vi "TimeLapse save images.vi"(7 "Logging queue":refnum<queue>, 8 "error in (no error)":errorcluster, 9 "Ch1-Green":i16[][](array[numeric]), 10 "Ch0-Red":i16[][](array[numeric]), 11 "Logging queue element":T1={"Imaging Protocol"=enum."Live Imaging", "Number of Trials"=0, "Frame Size"=512, "# Averaged frames"=0, "Dwell time (us)"=0.0, "Index of Z-plane"=0, "Timelapse?"=FALSE, "Logging process is active"=FALSE, "Speed logging enabled"=FALSE, "tdms file ref"=refnum, "path"=path "", "Trial Number"=0, "Expected # points acquired"=FALSE, "Manually stopped"=FALSE, "Ch0 data"=[], "Ch1 data"=[], "Last trial"=FALSE, "Points acquired"={"Ch0 last trial"=0, "Ch1 last trial"=0, "All trials"=0}} {"Frame Size" items=["100X100"=100, "128X128"=128, "200X200"=200, "256X256"=256, "512X512"=512, "1024x1024"=1024, "2048x2048"=2048]; "Dwell time (us)" format="%#.6g"}) -> (0 "error":errorcluster)   [LabVIEW 2013]
uses:
  Typedefs/Logging queue element.ctl
  Typedefs/Imaging Protocols enum.ctl
  Typedefs/Frame Size.ctl
  Typedefs/Acquired points count.ctl
  Typedefs/Channel Selector.ctl
  Typedefs/Top level VI states.ctl
  Global Variables/General Globals.vi
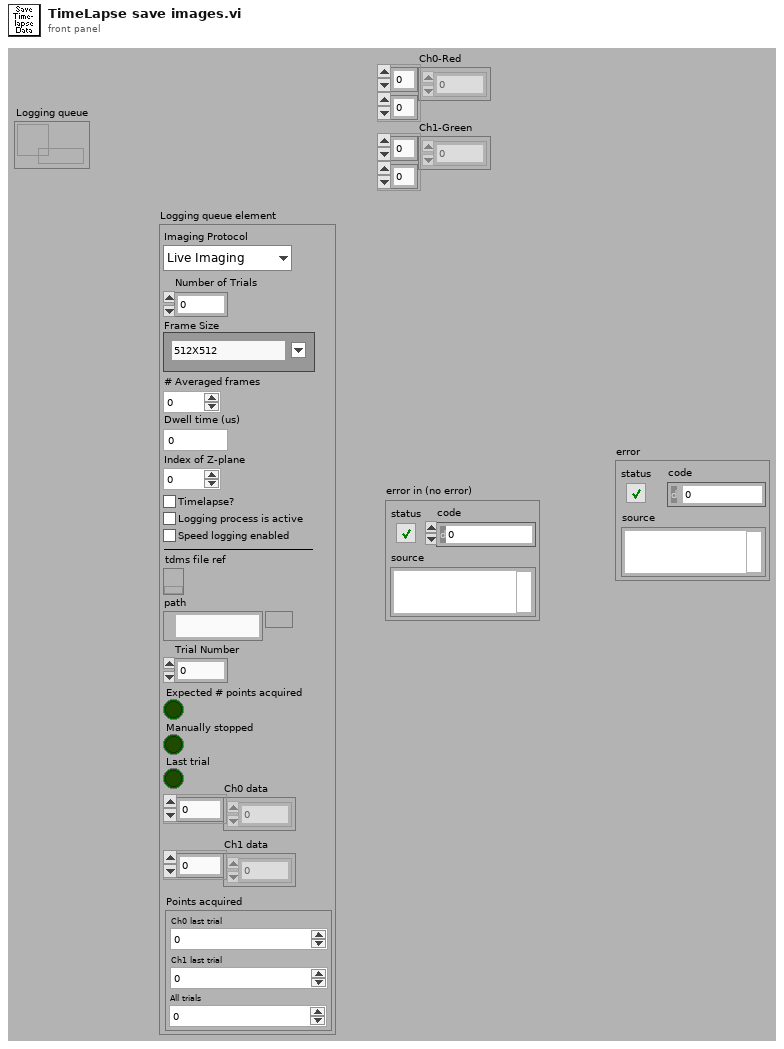
[diagram p1: front panel]
types:
  T1 = typedef "Logging queue element.ctl" = cluster{"Imaging Protocol":T2, "Number of Trials":u16, "Frame Size":T3, "# Averaged frames":u16, "Dwell time (us)":dbl, "Index of Z-plane":i32, "Timelapse?":bool, "Logging process is active":bool, "Speed logging enabled":bool, "tdms file ref":refnum<k34>, "path":path, "Trial Number":i32, "Expected # points acquired":bool, "Manually stopped":bool, "Ch0 data":u32[], "Ch1 data":u32[], "Last trial":bool, "Points acquired":T4}
  T2 = typedef "Imaging Protocols enum.ctl" = enum16{"AOL Z-Stack", "Motor Z Stack", "Functional Acquisition", "Single Plane Acquisition", "Volume Acquisition", "Live Imaging", "Live Plane Imaging", "Live Volume Imaging"}
  T3 = typedef "Frame Size.ctl" = u16
  T4 = typedef "Acquired points count.ctl" = cluster{"Ch0 last trial":u64, "Ch1 last trial":u64, "All trials":u64}
  T5 = typedef "Channel Selector.ctl" = enum16{"Red Channel", "Green Channel", "Blended"}
  T6 = typedef "Top level VI states.ctl" = enum16{"None", "Initialise UI", "<STACK PROTOCOL STATES>", "AOL Zstack-START", "AOL Zstack-STOP", "Motor Zstack-START", "Motor Zstack-STOP", "<ACQUISITION PROTOCOL STATES> ", "Functional Acquisition-START", "Functional Acquisition-STOP", "Single Plane Acquisition-START", "Single Plane Acquisition-STOP", "Volume Acquisition-START", "Volume Acquisition-STOP", "<LIVE IMAGING PROTOCOL STATES>", "Live Imaging-START", "Live Imaging-STOP", "Live Plane Imaging-START", "Live Plane Imaging-STOP", "Live Volume Imaging-START", "Live Volume Imaging-STOP", "EXIT"}
  T7 = typedef "AVI implementation enum.ctl" = enum16{"AVI1", "AVI2"}
  T8 = typedef "AVI Refs cluster.ctl" = cluster{"AVI2 path":path, "AVI 2 Refnum":T9, "New Image":T10, "error out":errorcluster, "Avi 1 Refnum":T11}
  T9 = typedef "IMAQ AVI2 Refnum.ctl" = refnum<k20>
  T10 = typedef "IMAQ Image.ctl" = refnum<image>
  T11 = typedef "AviRefnum.ctl" = refnum<k1>
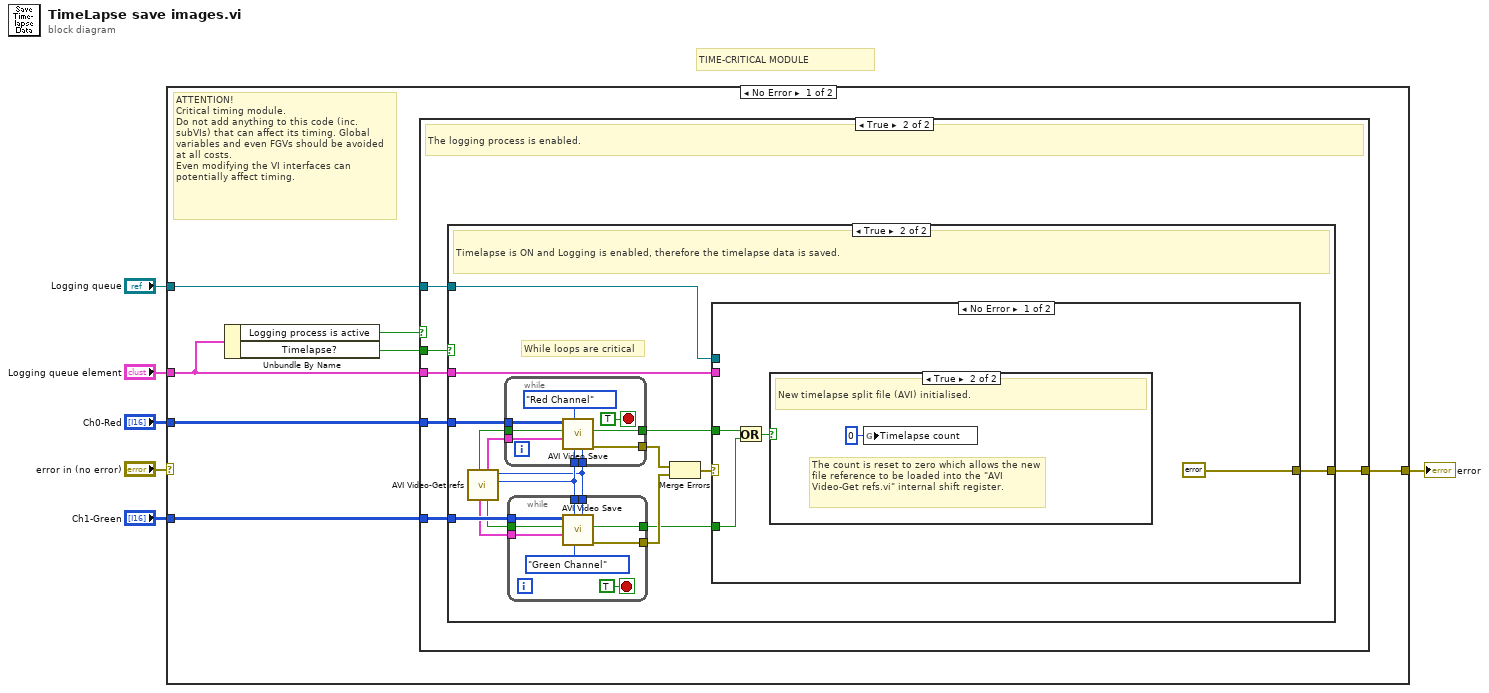
[diagram p0: block diagram]
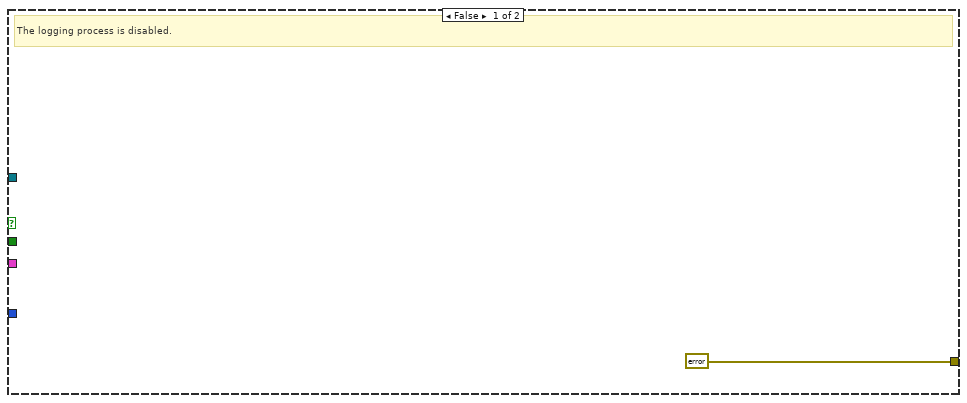
[diagram p2: hidden frame]
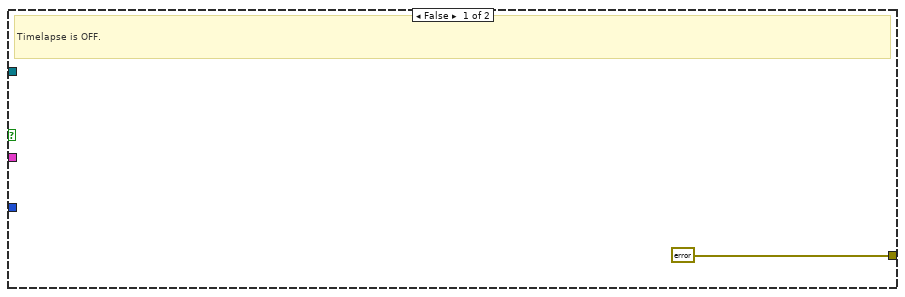
[diagram p3: hidden frame]
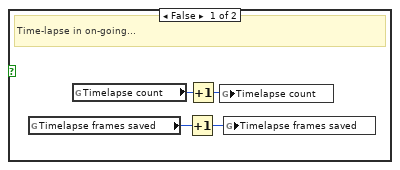
[diagram p4: hidden frame]
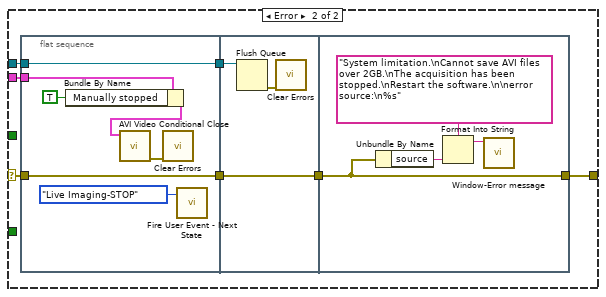
[diagram p5: hidden frame]
diagram:
  # "TIME-CRITICAL MODULE"
  n1 = case shown="No Error" "error in (no error)" {
    selector: "error in (no error)" -> [_ w86]
    tunnel: [w13 w86] -> w6
    tunnel: "Logging queue element" -> [w8 _]
    tunnel: "Ch0-Red" -> [w12 _]
    tunnel: "Ch1-Green" -> [w11 _]
    tunnel: "Logging queue" -> [w9 _]
    frame No Error {
      # "ATTENTION!\nCritical timing module.\nDo not add anything to this code (inc. subVIs) that can affect its timing. Global variables and even FGVs should be avoided at all costs.\nEven modifying the VI interfaces can potentially affect timing."
      n2 = Unbundle By Name(w8) -> ("Logging process is active"=w7:bool, "Timelapse?"=w10:bool)
      n3 = case shown="True" w7 {
        tunnel: [errorcluster {"status"=FALSE, "code"=0, "source"=""} ("error IO") w20] -> w13
        tunnel: w12 -> [_ w19]
        tunnel: w11 -> [_ w18]
        tunnel: w10 -> [_ w17]
        tunnel: w8 -> [_ w16]
        tunnel: w9 -> [_ w15]
        frame False {
          # "The logging process is disabled."
        }
        frame True {
          # "The logging process is enabled."
          n4 = case shown="True" w17 {
            tunnel: [errorcluster {"status"=FALSE, "code"=0, "source"=""} ("error IO") w26] -> w20
            tunnel: w19 -> [_ w35]
            tunnel: w18 -> [_ w34]
            tunnel: w16 -> [_ w28]
            tunnel: w15 -> [_ w27]
            frame False {
              # "Timelapse is OFF."
            }
            frame True {
              # "While loops are critical"
              # "Timelapse is ON and Logging is enabled, therefore the timelapse data is saved."
              n5 = call "AVI Video-Get refs.vi"() -> ("AVI mode"=w29:T7, "Frame Size"=w22:u32, "Green PMT is ON"=w31:bool, "Red AVI"=w32:T8, "Green AVI"=w30:T8, "Red PMT is ON"=w33:bool)  [unwired: 5 in, 1 out]
              n6 = while {
                tunnel: [w55] -> w36
                tunnel: w35 -> [w54]
                tunnel: w33 -> [w53]
                tunnel: w32 -> [w52]
                tunnel: w29 -> [w51]
                tunnel: [w49] -> w23
                tunnel: w22 -> [w48]
                stop <- TRUE stop-if-true
                n7 = call "AVI Video Save.vi"("Frame Size"=w48, "Channel"=Channel_Selector."Red Channel", "AVI mode"=w51, "AVI cluster"=w52, "PMT is ON?"=w53, "Image Pixels"=w54) -> ("error out"=w55:errorcluster, "New split file has just been initialised"=w49:bool)  [unwired: 4 in]
              }
              n8 = while {
                tunnel: [w46] -> w37
                tunnel: w34 -> [w45]
                tunnel: w31 -> [w44]
                tunnel: w30 -> [w43]
                tunnel: w29 -> [w42]
                tunnel: [w40] -> w24
                tunnel: w22 -> [w39]
                stop <- TRUE stop-if-true
                n9 = call "AVI Video Save.vi"("Frame Size"=w39, "Channel"=Channel_Selector."Green Channel", "AVI mode"=w42, "AVI cluster"=w43, "PMT is ON?"=w44, "Image Pixels"=w45) -> ("error out"=w46:errorcluster, "New split file has just been initialised"=w40:bool)  [unwired: 4 in]
              }
              n10 = Merge Errors(w36, w37) -> (w25:errorcluster)
              n11 = case shown="No Error" w25 {
                selector: w25 -> [_ w66]
                tunnel: w28 -> [_ w71]
                tunnel: w27 -> [_ w70]
                tunnel: [errorcluster {"status"=FALSE, "code"=0, "source"=""} ("error IO") w65] -> w26
                tunnel: w24 -> [w58 _]
                tunnel: w23 -> [w59 _]
                frame No Error {
                  n12 = Or(x=w59, y=w58) -> (x .or. y?=w57:bool)
                  n13 = case shown="True" w57 {
                    frame False {
                      # "Time-lapse in on-going..."
                      n14 = global read "General Globals.vi" "Timelapse frames saved"() -> (w61:u32)
                      n15 = global read "General Globals.vi" "Timelapse count"() -> (w62:u32)
                      n16 = Increment(x=w61) -> (x+1=w60:u32)
                      n17 = Increment(x=w62) -> (x+1=w63:u32)
                      n18 = global write "General Globals.vi" "Timelapse count"(w63) -> ()
                      n19 = global write "General Globals.vi" "Timelapse frames saved"(w60) -> ()
                    }
                    frame True {
                      # "The count is reset to zero which allows the new file reference to be loaded into the \"AVI Video-Get refs.vi\" internal shift register."
                      # "New timelapse split file (AVI) initialised."
                      n20 = global write "General Globals.vi" "Timelapse count"(u32 0 ("Timelapse count")) -> ()
                    }
                  }
                }
                frame Error {
                  n21 = flat-sequence {
                    tunnel: w71 -> [w77]
                    tunnel: [w74] -> w69
                    tunnel: w70 -> [w74]
                    tunnel: [w72] -> w67
                    tunnel: w66 -> [w72]
                    tunnel: w69 -> [w80]
                    tunnel: [w79] -> w68
                    tunnel: w67 -> [w79]
                    tunnel: w68 -> [w82]
                    tunnel: [w82] -> w65
                    frame #0 {
                      n22 = Bundle By Name(cluster=w77, "Manually stopped"=TRUE) -> (w75:T1)
                      n23 = call "AVI Video Conditional Close.vi"("Logging queue element in"=w75) -> ("error out"=w78:errorcluster)  [unwired: 10 in]
                      n24 = call <vilib>:"Clear Errors.vi"("error in (no error)"=w78) -> ()  [unwired: 6 in, 1 out]
                      n25 = call "Fire User Event - Next State.vi"("\"UI Handler loop\" case to execute"=Top_level_VI_states."Live Imaging-STOP" ("event data / imaging mode")) -> ()  [unwired: 10 in, 1 out]
                    }
                    frame #1 {
                      n26 = Flush Queue(queue=w80) -> (error out=w81:errorcluster)  [unwired: 1 in, 2 out]
                      n27 = call <vilib>:"Clear Errors.vi"("error in (no error)"=w81) -> ()  [unwired: 6 in, 1 out]
                    }
                    frame #2 {
                      n28 = Unbundle By Name(w82) -> ("source"=w84:string)
                      n29 = Format Into String(format string="System limitation.\nCannot save AVI files over 2GB.\nThe acquisition has been stopped.\nRestart the software.\n\nerror source:\n%s", w84) -> (resulting string=w83:string)  [unwired: 2 in, 1 out]
                      n30 = call "Window-Error message.vi"("Message"=w83) -> ()  [unwired: 10 in, 1 out]
                    }
                  }
                }
              }
            }
          }
        }
      }
    }
    frame Error {
    }
  }
  "error" <- w6
